vi "FirmwareForPython.vi"() -> ()   [LabVIEW 2018]
uses:
  <vilib>/rvi/Emulation/niFpgaGetClockAttributes.vi
  <vilib>/rvi/Emulation/niFpgaSctlEmulationGetInTimedLoop.vi
  <vilib>/rvi/Emulation/niFpgaEmulationReportErrorSimple.vi
  <vilib>/rvi/Emulation/niFpgaEmulationIsFPGAContextNoSignature.vi
  <vilib>/rvi/errors/niFpgaSetErrorForExecOnDevCompSimple.vi
  <vilib>/rvi/eio/common/nirviEmuReportErrorAndStop.vi
  <vilib>/rvi/DataTransferAndStorage/Container/Common/niFpgaContainerGetUniqueNameForEmu.vi
  <vilib>/rvi/FIFO/Fifo_Resource/nirvififoEmulationSetSize.vi
  <vilib>/rvi/FIFO/Fifo_Resource/nirviFifoEmulationQueueMgr.vi
  <instcachedir>/0/nirviFifoEmulationQueueMgr_E5CAEC123FF24DC58D834DCA3CDAA9B5.lvgen/nirviFifoEmulationQueueMgr_E5CAEC123FF24DC58D834DCA3CDAA9B5_001.vi
  <vilib>/Utility/error.llb/Clear Errors.vi
  <vilib>/rvi/FIFO/Fifo_Resource/nirvififoEmulationCreateLock.vi
  <vilib>/rvi/Emulation/niFpgaProcessEmulError.vi
  <vilib>/rvi/FIFO/Fifo_Resource/nirvififoEmulationObtainLock.vi
  <vilib>/rvi/FIFO/Fifo_Resource/nirvififoEmulationReleaseLock.vi
  <vilib>/rvi/occurrence/nirviWaitOnOccurrenceBase.vi
  <vilib>/rvi/errors/nirviReportUnexpectedCaseInternalError.vi
  <vilib>/rvi/errors/nirviReportUnexpectedCaseInternalError (U32).vi
  <vilib>/rvi/interface/RandomDataEmulation/niFpgaRandomDataHandleErrors.vi
  <vilib>/rvi/Emulation/niFpgaCriticalErrorInLSC.vi
  <vilib>/rvi/eio/common/nirviEmuTemplateMethod_errors.vi
  <vilib>/rvi/FIFO/Fifo_Resource/nirvififoEmulationDetermineInputValidOut.vi
  <vilib>/rvi/DataTransferAndStorage/Container/XNode/niFpgaContainer.xnode
  <vilib>/rvi/FIFO/Fifo_Resource/nirvififoEmulationRead.vi
  <vilib>/rvi/interface/RandomDataEmulation/nirviRandomDataFpgaReadWriteTemplate.vi
  <vilib>/eio/EIONode/EIONode.xnode
  <vilib>/rvi/FIFO/Fifo_Resource/nirvififoEmulationWrite.vi
panel:
  in  "DIO14-IN":bool
  in  "DIO1-IN":bool
  in  "DIO13-IN":bool
  in  "DIO11-IN":bool
  in  "DIO2-IN":bool
  in  "DIO12-IN":bool
  in  "DIO15-IN":bool
  in  "DIO10-IN":bool
  in  "DIO8-IN":bool
  in  "DIO9-IN":bool
  in  "DIO7-IN":bool
  in  "DIO6-IN":bool
  in  "DIO5-IN":bool
  in  "DIO4-IN":bool
  in  "DIO3-IN":bool
  in  "DIO0-IN":bool
  out "DI15":bool
  out "DI14":bool
  out "DI13":bool
  out "DI12":bool
  out "DI11":bool
  out "DI10":bool
  out "DI9":bool
  out "DI8":bool
  out "DI7":bool
  out "DI6":bool
  out "DI5":bool
  out "DI4":bool
  out "DI3":bool
  out "DI2":bool
  out "DI1":bool
  in  "DO15":bool
  in  "DO14":bool
  in  "DO13":bool
  in  "DO12":bool
  in  "DO11":bool
  in  "DO10":bool
  in  "DO9":bool
  in  "DO8":bool
  in  "DO7":bool
  in  "DO6":bool
  in  "DO5":bool
  in  "DO4":bool
  in  "DO3":bool
  in  "DO2":bool
  in  "DO1":bool
  in  "DO0":bool
  out "DI0":bool
  in  "Sampling-DIO":u32 caption="Count(Ticks)"
  out "Timeout-DIO":bool
  in  "AO1":i16
  in  "AO3":i16
  in  "AO7":i16
  in  "AO2":i16
  in  "AO6":i16
  in  "AO4":i16
  in  "AO5":i16
  in  "AO0":i16
  in  "Sampling-AO":u32 caption="Count(Ticks)"
  out "Timeout-AO":bool
  in  "Bonus1channel":i16
  out "Bonus1-FIFO-Timeout":bool
  out "Acquisition\nTimeout-Bonus1":bool
  in  "Sampling-Bonus1":u32 caption="Count(Ticks)"
  out "DC-FIFO-Timeout":bool
  in  "DCchannel":i16
  out "Acquisition\nTimeout-DC":bool
  in  "Sampling-DC":u32 caption="Count(Ticks)"
  in  "Zchannel":i16
  in  "Ychannel":i16
  in  "Xchannel":i16
  out "Z-tmeout":bool
  out "X-timeout":bool
  out "Y-timeout":bool
  out "Acquisition\nTimeout":bool
  in  "Sampling":u32 caption="Count(Ticks)"
  out "data FIFO":bool
  out "FIFO Y":bool
  out "FIFO X":bool
  out "FIFO Z-balanced":bool
  out "FIFO-acquisition":bool
  in  "Interleaving \nSampling":u32 caption="Count(Ticks)"
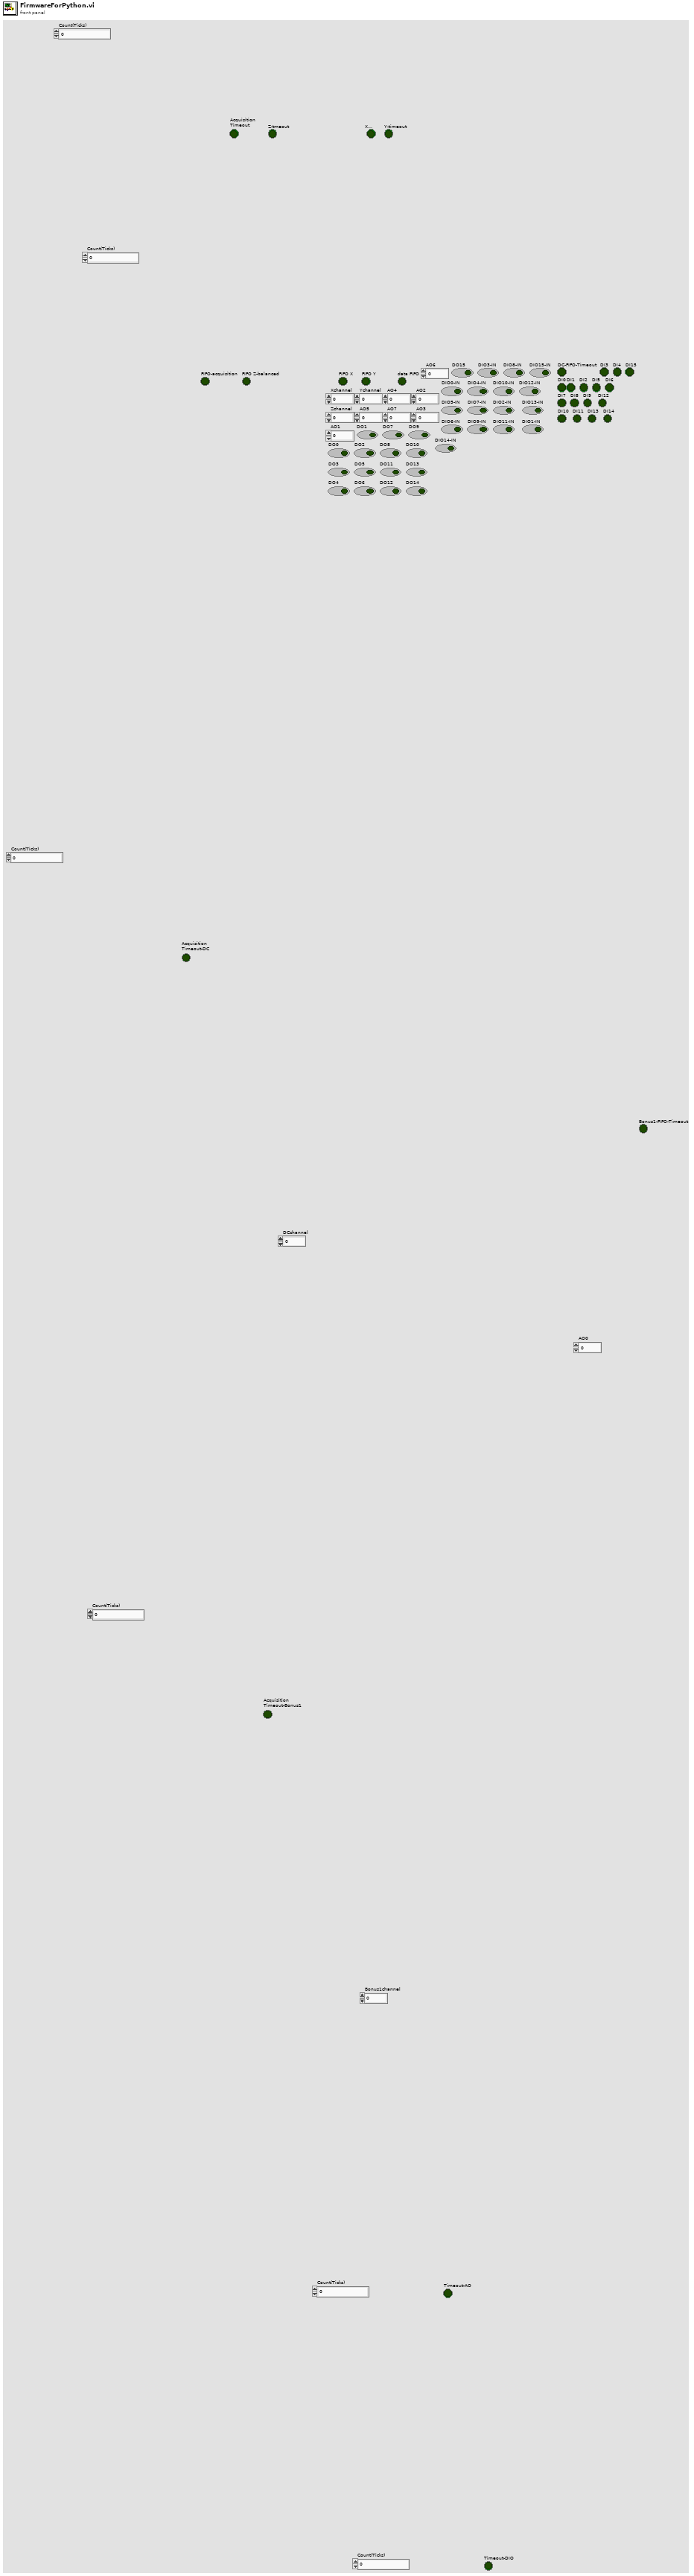
[diagram p1: front panel]
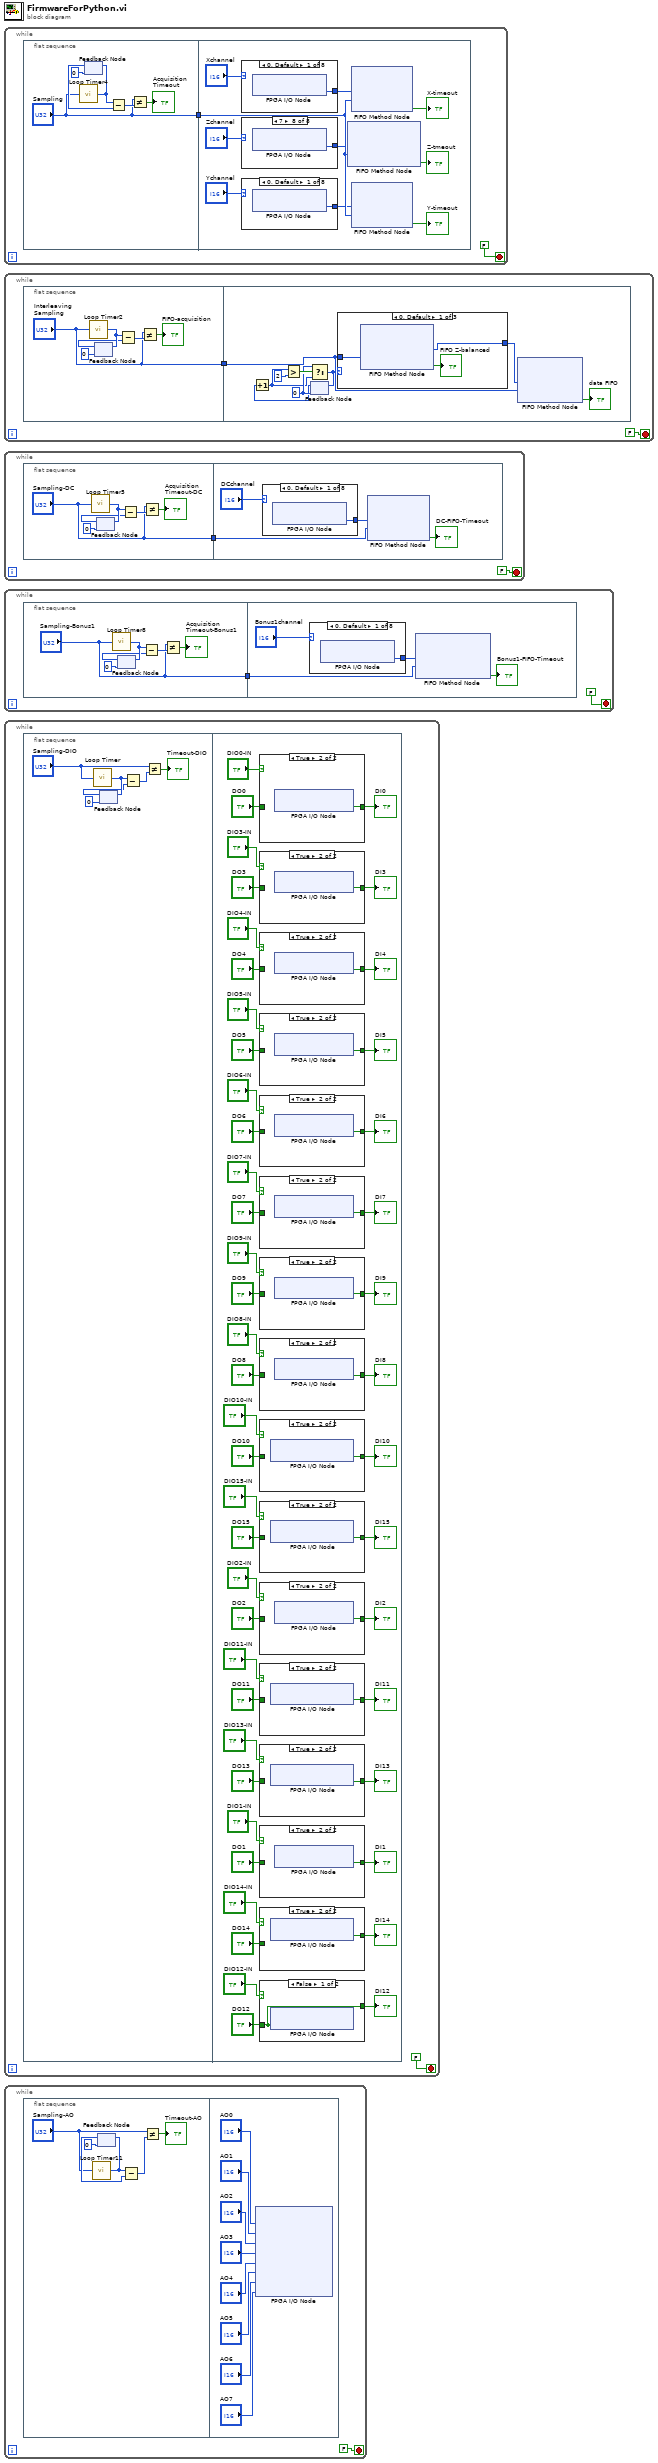
[diagram p0: block diagram]
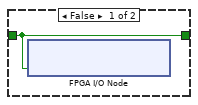
[diagram p2: hidden frame]
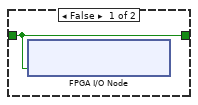
[diagram p3: hidden frame]
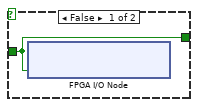
[diagram p4: hidden frame]
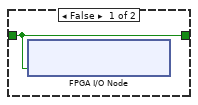
[diagram p5: hidden frame]
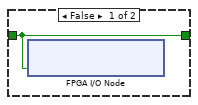
[diagram p6: hidden frame]
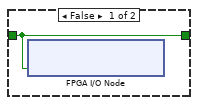
[diagram p7: hidden frame]
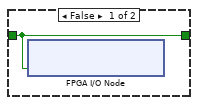
[diagram p8: hidden frame]
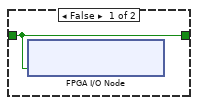
[diagram p9: hidden frame]
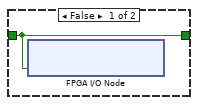
[diagram p10: hidden frame]
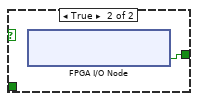
[diagram p11: hidden frame]
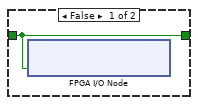
[diagram p12: hidden frame]
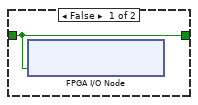
[diagram p13: hidden frame]
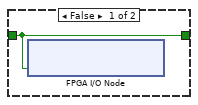
[diagram p14: hidden frame]
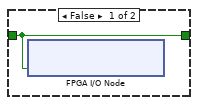
[diagram p15: hidden frame]
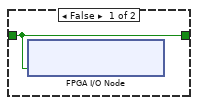
[diagram p16: hidden frame]
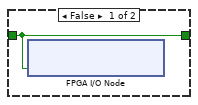
[diagram p17: hidden frame]
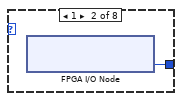
[diagram p18: hidden frame]
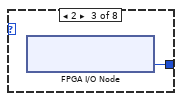
[diagram p19: hidden frame]
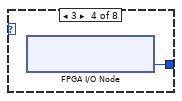
[diagram p20: hidden frame]
diagram:
  n1 = while {
    stop <- FALSE stop-if-true
    n2 = flat-sequence {
      tunnel: ["Sampling"] -> w1
      tunnel: w1 -> [w15]
      frame #0 {
        n3 = call "Loop Timer4"("Count(Ticks)"="Sampling") -> ("Tick Count(Ticks)"=w7:u32)
        n4 = feedback-in #1(w7) -> ()
        n5 = feedback #1(u32 0 ("Tick Count(Ticks)")) -> (w6:u32)
        n6 = Subtract(x=w7, y=w6) -> (x-y=w5:u32)
        n7 = Not Equal?(x="Sampling", y=w5) -> (x != y?=→"Acquisition\nTimeout":bool)
      }
      frame #1 {
        n8 = case shown="0, Default" "Xchannel" {
          tunnel: [w35 w36 w37 w38 w39 w40 w41 w42] -> w13
          frame 0, Default {
            n9 = xnode "FPGA I/O Node"() -> ("Connector0/AI0"=w35:i16)  [unwired: 1 in, 1 out]
          }
          frame 1 {
            n10 = xnode "FPGA I/O Node"() -> ("Connector0/AI1"=w36:i16)  [unwired: 1 in, 1 out]
          }
          frame 2 {
            n11 = xnode "FPGA I/O Node"() -> ("Connector0/AI2"=w37:i16)  [unwired: 1 in, 1 out]
          }
          frame 3 {
            n12 = xnode "FPGA I/O Node"() -> ("Connector0/AI3"=w38:i16)  [unwired: 1 in, 1 out]
          }
          frame 4 {
            n13 = xnode "FPGA I/O Node"() -> ("Connector0/AI4"=w39:i16)  [unwired: 1 in, 1 out]
          }
          frame 5 {
            n14 = xnode "FPGA I/O Node"() -> ("Connector0/AI5"=w40:i16)  [unwired: 1 in, 1 out]
          }
          frame 6 {
            n15 = xnode "FPGA I/O Node"() -> ("Connector0/AI6"=w41:i16)  [unwired: 1 in, 1 out]
          }
          frame 7 {
            n16 = xnode "FPGA I/O Node"() -> ("Connector0/AI7"=w42:i16)  [unwired: 1 in, 1 out]
          }
        }
        n17 = case shown="7" "Zchannel" {
          tunnel: [w19 w20 w21 w22 w23 w24 w25 w26] -> w9
          frame 0, Default {
            n18 = xnode "FPGA I/O Node"() -> ("Connector0/AI0"=w19:i16)  [unwired: 1 in, 1 out]
          }
          frame 1 {
            n19 = xnode "FPGA I/O Node"() -> ("Connector0/AI1"=w20:i16)  [unwired: 1 in, 1 out]
          }
          frame 2 {
            n20 = xnode "FPGA I/O Node"() -> ("Connector0/AI2"=w21:i16)  [unwired: 1 in, 1 out]
          }
          frame 3 {
            n21 = xnode "FPGA I/O Node"() -> ("Connector0/AI3"=w22:i16)  [unwired: 1 in, 1 out]
          }
          frame 4 {
            n22 = xnode "FPGA I/O Node"() -> ("Connector0/AI4"=w23:i16)  [unwired: 1 in, 1 out]
          }
          frame 5 {
            n23 = xnode "FPGA I/O Node"() -> ("Connector0/AI5"=w24:i16)  [unwired: 1 in, 1 out]
          }
          frame 6 {
            n24 = xnode "FPGA I/O Node"() -> ("Connector0/AI6"=w25:i16)  [unwired: 1 in, 1 out]
          }
          frame 7 {
            n25 = xnode "FPGA I/O Node"() -> ("Connector0/AI7"=w26:i16)  [unwired: 1 in, 1 out]
          }
        }
        n26 = case shown="0, Default" "Ychannel" {
          tunnel: [w27 w28 w29 w30 w31 w32 w33 w34] -> w11
          frame 0, Default {
            n27 = xnode "FPGA I/O Node"() -> ("Connector0/AI0"=w27:i16)  [unwired: 1 in, 1 out]
          }
          frame 1 {
            n28 = xnode "FPGA I/O Node"() -> ("Connector0/AI1"=w28:i16)  [unwired: 1 in, 1 out]
          }
          frame 2 {
            n29 = xnode "FPGA I/O Node"() -> ("Connector0/AI2"=w29:i16)  [unwired: 1 in, 1 out]
          }
          frame 3 {
            n30 = xnode "FPGA I/O Node"() -> ("Connector0/AI3"=w30:i16)  [unwired: 1 in, 1 out]
          }
          frame 4 {
            n31 = xnode "FPGA I/O Node"() -> ("Connector0/AI4"=w31:i16)  [unwired: 1 in, 1 out]
          }
          frame 5 {
            n32 = xnode "FPGA I/O Node"() -> ("Connector0/AI5"=w32:i16)  [unwired: 1 in, 1 out]
          }
          frame 6 {
            n33 = xnode "FPGA I/O Node"() -> ("Connector0/AI6"=w33:i16)  [unwired: 1 in, 1 out]
          }
          frame 7 {
            n34 = xnode "FPGA I/O Node"() -> ("Connector0/AI7"=w34:i16)  [unwired: 1 in, 1 out]
          }
        }
        n35 = xnode ("FIFO Method Node")("Element"=w9, "Timeout"=w15) -> ("Timed Out?"=→"Z-tmeout":bool)  [unwired: 1 in, 1 out]
        n36 = xnode ("FIFO Method Node")("Element"=w13, "Timeout"=w15) -> ("Timed Out?"=→"X-timeout":bool)  [unwired: 1 in, 1 out]
        n37 = xnode ("FIFO Method Node")("Element"=w11, "Timeout"=w15) -> ("Timed Out?"=→"Y-timeout":bool)  [unwired: 1 in, 1 out]
      }
    }
  }
  n38 = while {
    stop <- FALSE stop-if-true
    n39 = flat-sequence {
      tunnel: ["Interleaving \nSampling"] -> w43
      tunnel: w43 -> [w58]
      frame #0 {
        n40 = call "Loop Timer2"("Count(Ticks)"="Interleaving \nSampling") -> ("Tick Count(Ticks)"=w49:u32)
        n41 = feedback-in #2(w49) -> ()
        n42 = feedback #2(u32 0 ("Tick Count(Ticks)")) -> (w48:u32)
        n43 = Subtract(x=w49, y=w48) -> (x-y=w47:u32)
        n44 = Not Equal?(x="Interleaving \nSampling", y=w47) -> (x != y?=→"FIFO-acquisition":bool)
      }
      frame #1 {
        w54 = i16 0
        n45 = feedback #3(w54) -> (w53:i16)
        n46 = Increment(x=w53) -> (x+1=w51:i16)
        n47 = Greater?(x=w51, y=i16 2) -> (0:w55:bool)
        n48 = Select(t=w54, s=w55, f=w51) -> (s? t:f=w52:i16)
        n49 = feedback-in #3(w52) -> ()
        n50 = case shown="0, Default" w52 {
          tunnel: w58 -> [w62 w63 w67]
          tunnel: [w60 w65 w66] -> w57
          frame 0, Default {
            n51 = xnode ("FIFO Method Node")("Timeout"=w62) -> ("Element"=w60:i16, "Timed Out?"=→"FIFO Z-balanced":bool)  [unwired: 1 in, 1 out]
          }
          frame 1 {
            n52 = xnode ("FIFO Method Node")("Timeout"=w63) -> ("Element"=w65:i16, "Timed Out?"=→"FIFO X":bool)  [unwired: 1 in, 1 out]
          }
          frame 2 {
            n53 = xnode ("FIFO Method Node")("Timeout"=w67) -> ("Element"=w66:i16, "Timed Out?"=→"FIFO Y":bool)  [unwired: 1 in, 1 out]
          }
        }
        n54 = xnode ("FIFO Method Node")("Element"=w57, "Timeout"=w58) -> ("Timed Out?"=→"data FIFO":bool)  [unwired: 1 in, 1 out]
      }
    }
  }
  n55 = while {
    stop <- FALSE stop-if-true
    n56 = flat-sequence {
      tunnel: ["Sampling-DC"] -> w69
      tunnel: w69 -> [w77]
      frame #0 {
        n57 = call "Loop Timer5"("Count(Ticks)"="Sampling-DC") -> ("Tick Count(Ticks)"=w75:u32)
        n58 = feedback-in #4(w75) -> ()
        n59 = feedback #4(u32 0 ("Tick Count(Ticks)")) -> (w74:u32)
        n60 = Subtract(x=w75, y=w74) -> (x-y=w73:u32)
        n61 = Not Equal?(x="Sampling-DC", y=w73) -> (x != y?=→"Acquisition\nTimeout-DC":bool)
      }
      frame #1 {
        n62 = case shown="0, Default" "DCchannel" {
          tunnel: [w81 w82 w83 w84 w85 w86 w87 w88] -> w78
          frame 0, Default {
            n63 = xnode "FPGA I/O Node"() -> ("Connector0/AI0"=w81:i16)  [unwired: 1 in, 1 out]
          }
          frame 1 {
            n64 = xnode "FPGA I/O Node"() -> ("Connector0/AI1"=w82:i16)  [unwired: 1 in, 1 out]
          }
          frame 2 {
            n65 = xnode "FPGA I/O Node"() -> ("Connector0/AI2"=w83:i16)  [unwired: 1 in, 1 out]
          }
          frame 3 {
            n66 = xnode "FPGA I/O Node"() -> ("Connector0/AI3"=w84:i16)  [unwired: 1 in, 1 out]
          }
          frame 4 {
            n67 = xnode "FPGA I/O Node"() -> ("Connector0/AI4"=w85:i16)  [unwired: 1 in, 1 out]
          }
          frame 5 {
            n68 = xnode "FPGA I/O Node"() -> ("Connector0/AI5"=w86:i16)  [unwired: 1 in, 1 out]
          }
          frame 6 {
            n69 = xnode "FPGA I/O Node"() -> ("Connector0/AI6"=w87:i16)  [unwired: 1 in, 1 out]
          }
          frame 7 {
            n70 = xnode "FPGA I/O Node"() -> ("Connector0/AI7"=w88:i16)  [unwired: 1 in, 1 out]
          }
        }
        n71 = xnode ("FIFO Method Node")("Element"=w78, "Timeout"=w77) -> ("Timed Out?"=→"DC-FIFO-Timeout":bool)  [unwired: 1 in, 1 out]
      }
    }
  }
  n72 = while {
    stop <- FALSE stop-if-true
    n73 = flat-sequence {
      tunnel: ["Sampling-Bonus1"] -> w89
      tunnel: w89 -> [w98]
      frame #0 {
        n74 = call "Loop Timer8"("Count(Ticks)"="Sampling-Bonus1") -> ("Tick Count(Ticks)"=w95:u32)
        n75 = feedback-in #5(w95) -> ()
        n76 = feedback #5(u32 0 ("Tick Count(Ticks)")) -> (w94:u32)
        n77 = Subtract(x=w95, y=w94) -> (x-y=w93:u32)
        n78 = Not Equal?(x="Sampling-Bonus1", y=w93) -> (x != y?=→"Acquisition\nTimeout-Bonus1":bool)
      }
      frame #1 {
        n79 = case shown="0, Default" "Bonus1channel" {
          tunnel: [w101 w102 w103 w104 w105 w106 w107 w108] -> w99
          frame 0, Default {
            n80 = xnode "FPGA I/O Node"() -> ("Connector0/AI0"=w101:i16)  [unwired: 1 in, 1 out]
          }
          frame 1 {
            n81 = xnode "FPGA I/O Node"() -> ("Connector0/AI1"=w102:i16)  [unwired: 1 in, 1 out]
          }
          frame 2 {
            n82 = xnode "FPGA I/O Node"() -> ("Connector0/AI2"=w103:i16)  [unwired: 1 in, 1 out]
          }
          frame 3 {
            n83 = xnode "FPGA I/O Node"() -> ("Connector0/AI3"=w104:i16)  [unwired: 1 in, 1 out]
          }
          frame 4 {
            n84 = xnode "FPGA I/O Node"() -> ("Connector0/AI4"=w105:i16)  [unwired: 1 in, 1 out]
          }
          frame 5 {
            n85 = xnode "FPGA I/O Node"() -> ("Connector0/AI5"=w106:i16)  [unwired: 1 in, 1 out]
          }
          frame 6 {
            n86 = xnode "FPGA I/O Node"() -> ("Connector0/AI6"=w107:i16)  [unwired: 1 in, 1 out]
          }
          frame 7 {
            n87 = xnode "FPGA I/O Node"() -> ("Connector0/AI7"=w108:i16)  [unwired: 1 in, 1 out]
          }
        }
        n88 = xnode ("FIFO Method Node")("Element"=w99, "Timeout"=w98) -> ("Timed Out?"=→"Bonus1-FIFO-Timeout":bool)  [unwired: 1 in, 1 out]
      }
    }
  }
  n89 = while {
    stop <- FALSE stop-if-true
    n90 = flat-sequence {
      frame #0 {
        n91 = call "Loop Timer"("Count(Ticks)"="Sampling-DIO") -> ("Tick Count(Ticks)"=w114:u32)
        n92 = feedback-in #6(w114) -> ()
        n93 = feedback #6(u32 0 ("Tick Count(Ticks)")) -> (w113:u32)
        n94 = Subtract(x=w114, y=w113) -> (x-y=w112:u32)
        n95 = Not Equal?(x="Sampling-DIO", y=w112) -> (x != y?=→"Timeout-DIO":bool)
      }
      frame #1 {
        n96 = case shown="True" "DIO0-IN" {
          tunnel: [w194 w195] -> w163
          tunnel: "DO0" -> [w194 _]
          frame False {
            n97 = xnode "FPGA I/O Node"("Connector0/DIO0"=w194) -> ()  [unwired: 1 in, 1 out]
          }
          frame True {
            n98 = xnode "FPGA I/O Node"() -> ("Connector0/DIO0"=w195:bool)  [unwired: 1 in, 1 out]
          }
        }
        "DI0" <- w163
        n99 = case shown="True" "DIO3-IN" {
          tunnel: [w192 w193] -> w156
          tunnel: "DO3" -> [w192 _]
          frame False {
            n100 = xnode "FPGA I/O Node"("Connector0/DIO3"=w192) -> ()  [unwired: 1 in, 1 out]
          }
          frame True {
            n101 = xnode "FPGA I/O Node"() -> ("Connector0/DIO3"=w193:bool)  [unwired: 1 in, 1 out]
          }
        }
        "DI3" <- w156
        n102 = case shown="True" "DIO4-IN" {
          tunnel: [w176 w177] -> w154
          tunnel: "DO4" -> [w176 _]
          frame False {
            n103 = xnode "FPGA I/O Node"("Connector0/DIO4"=w176) -> ()  [unwired: 1 in, 1 out]
          }
          frame True {
            n104 = xnode "FPGA I/O Node"() -> ("Connector0/DIO4"=w177:bool)  [unwired: 1 in, 1 out]
          }
        }
        "DI4" <- w154
        n105 = case shown="True" "DIO5-IN" {
          tunnel: [w190 w191] -> w152
          tunnel: "DO5" -> [w190 _]
          frame False {
            n106 = xnode "FPGA I/O Node"("Connector0/DIO5"=w190) -> ()  [unwired: 1 in, 1 out]
          }
          frame True {
            n107 = xnode "FPGA I/O Node"() -> ("Connector0/DIO5"=w191:bool)  [unwired: 1 in, 1 out]
          }
        }
        "DI5" <- w152
        n108 = case shown="True" "DIO6-IN" {
          tunnel: [w174 w175] -> w150
          tunnel: "DO6" -> [w174 _]
          frame False {
            n109 = xnode "FPGA I/O Node"("Connector0/DIO6"=w174) -> ()  [unwired: 1 in, 1 out]
          }
          frame True {
            n110 = xnode "FPGA I/O Node"() -> ("Connector0/DIO6"=w175:bool)  [unwired: 1 in, 1 out]
          }
        }
        "DI6" <- w150
        n111 = case shown="True" "DIO7-IN" {
          tunnel: [w188 w189] -> w148
          tunnel: "DO7" -> [w188 _]
          frame False {
            n112 = xnode "FPGA I/O Node"("Connector0/DIO7"=w188) -> ()  [unwired: 1 in, 1 out]
          }
          frame True {
            n113 = xnode "FPGA I/O Node"() -> ("Connector0/DIO7"=w189:bool)  [unwired: 1 in, 1 out]
          }
        }
        "DI7" <- w148
        n114 = case shown="True" "DIO9-IN" {
          tunnel: [w172 w173] -> w144
          tunnel: "DO9" -> [w172 _]
          frame False {
            n115 = xnode "FPGA I/O Node"("Connector0/DIO9"=w172) -> ()  [unwired: 1 in, 1 out]
          }
          frame True {
            n116 = xnode "FPGA I/O Node"() -> ("Connector0/DIO9"=w173:bool)  [unwired: 1 in, 1 out]
          }
        }
        "DI9" <- w144
        n117 = case shown="True" "DIO8-IN" {
          tunnel: [w186 w187] -> w146
          tunnel: "DO8" -> [w186 _]
          frame False {
            n118 = xnode "FPGA I/O Node"("Connector0/DIO8"=w186) -> ()  [unwired: 1 in, 1 out]
          }
          frame True {
            n119 = xnode "FPGA I/O Node"() -> ("Connector0/DIO8"=w187:bool)  [unwired: 1 in, 1 out]
          }
        }
        "DI8" <- w146
        n120 = case shown="True" "DIO10-IN" {
          tunnel: [w184 w185] -> w142
          tunnel: "DO10" -> [w184 _]
          frame False {
            n121 = xnode "FPGA I/O Node"("Connector0/DIO10"=w184) -> ()  [unwired: 1 in, 1 out]
          }
          frame True {
            n122 = xnode "FPGA I/O Node"() -> ("Connector0/DIO10"=w185:bool)  [unwired: 1 in, 1 out]
          }
        }
        "DI10" <- w142
        n123 = case shown="True" "DIO15-IN" {
          tunnel: [w166 w167] -> w137
          tunnel: "DO15" -> [w166 _]
          frame False {
            n124 = xnode "FPGA I/O Node"("Connector0/DIO15"=w166) -> ()  [unwired: 1 in, 1 out]
          }
          frame True {
            n125 = xnode "FPGA I/O Node"() -> ("Connector0/DIO15"=w167:bool)  [unwired: 1 in, 1 out]
          }
        }
        "DI15" <- w137
        n126 = case shown="True" "DIO2-IN" {
          tunnel: [w178 w179] -> w158
          tunnel: "DO2" -> [w178 _]
          frame False {
            n127 = xnode "FPGA I/O Node"("Connector0/DIO2"=w178) -> ()  [unwired: 1 in, 1 out]
          }
          frame True {
            n128 = xnode "FPGA I/O Node"() -> ("Connector0/DIO2"=w179:bool)  [unwired: 1 in, 1 out]
          }
        }
        "DI2" <- w158
        n129 = case shown="True" "DIO11-IN" {
          tunnel: [w170 w171] -> w134
          tunnel: "DO11" -> [w170 _]
          frame False {
            n130 = xnode "FPGA I/O Node"("Connector0/DIO11"=w170) -> ()  [unwired: 1 in, 1 out]
          }
          frame True {
            n131 = xnode "FPGA I/O Node"() -> ("Connector0/DIO11"=w171:bool)  [unwired: 1 in, 1 out]
          }
        }
        "DI11" <- w134
        n132 = case shown="True" "DIO13-IN" {
          tunnel: [w164 w165] -> w140
          tunnel: "DO13" -> [w164 _]
          frame False {
            n133 = xnode "FPGA I/O Node"("Connector0/DIO13"=w164) -> ()  [unwired: 1 in, 1 out]
          }
          frame True {
            n134 = xnode "FPGA I/O Node"() -> ("Connector0/DIO13"=w165:bool)  [unwired: 1 in, 1 out]
          }
        }
        "DI13" <- w140
        n135 = case shown="True" "DIO1-IN" {
          tunnel: [w180 w181] -> w160
          tunnel: "DO1" -> [w180 _]
          frame False {
            n136 = xnode "FPGA I/O Node"("Connector0/DIO1"=w180) -> ()  [unwired: 1 in, 1 out]
          }
          frame True {
            n137 = xnode "FPGA I/O Node"() -> ("Connector0/DIO1"=w181:bool)  [unwired: 1 in, 1 out]
          }
        }
        "DI1" <- w160
        n138 = case shown="True" "DIO14-IN" {
          tunnel: [w168 w169] -> w135
          tunnel: "DO14" -> [w168 _]
          frame False {
            n139 = xnode "FPGA I/O Node"("Connector0/DIO14"=w168) -> ()  [unwired: 1 in, 1 out]
          }
          frame True {
            n140 = xnode "FPGA I/O Node"() -> ("Connector0/DIO14"=w169:bool)  [unwired: 1 in, 1 out]
          }
        }
        "DI14" <- w135
        n141 = case shown="False" "DIO12-IN" {
          tunnel: [w182 w183] -> w116
          tunnel: "DO12" -> [w182 _]
          frame False {
            n142 = xnode "FPGA I/O Node"("Connector0/DIO12"=w182) -> ()  [unwired: 1 in, 1 out]
          }
          frame True {
            n143 = xnode "FPGA I/O Node"() -> ("Connector0/DIO12"=w183:bool)  [unwired: 1 in, 1 out]
          }
        }
        "DI12" <- w116
      }
    }
  }
  n144 = while {
    stop <- FALSE stop-if-true
    n145 = flat-sequence {
      frame #0 {
        n146 = call "Loop Timer11"("Count(Ticks)"="Sampling-AO") -> ("Tick Count(Ticks)"=w201:u32)
        n147 = feedback-in #7(w201) -> ()
        n148 = feedback #7(u32 0 ("Tick Count(Ticks)")) -> (w200:u32)
        n149 = Subtract(x=w201, y=w200) -> (x-y=w199:u32)
        n150 = Not Equal?(x="Sampling-AO", y=w199) -> (x != y?=→"Timeout-AO":bool)
      }
      frame #1 {
        n151 = xnode "FPGA I/O Node"("Connector0/AO0"="AO0", "Connector0/AO1"="AO1", "Connector0/AO2"="AO2", "Connector0/AO3"="AO3", "Connector0/AO4"="AO4", "Connector0/AO5"="AO5", "Connector0/AO6"="AO6", "Connector0/AO7"="AO7") -> ()  [unwired: 8 in, 8 out]
      }
    }
  }
